vi "古田户外一体站流程自动启动.vi"(11 "参数":T1={"是否启用仪器"=FALSE, "CODMn"={"启动测量模式"={"测量模式"=enum."水样测量"}, "确定按钮"=TRUE}}) -> ()   [LabVIEW 2016, in "PLC.lvlib"]
uses:
  PLC.lvlib
panel:
  out "枚举":enum16{"初始化", "采配水启动", "等待", "配水", "排水", "结束"}(ring)
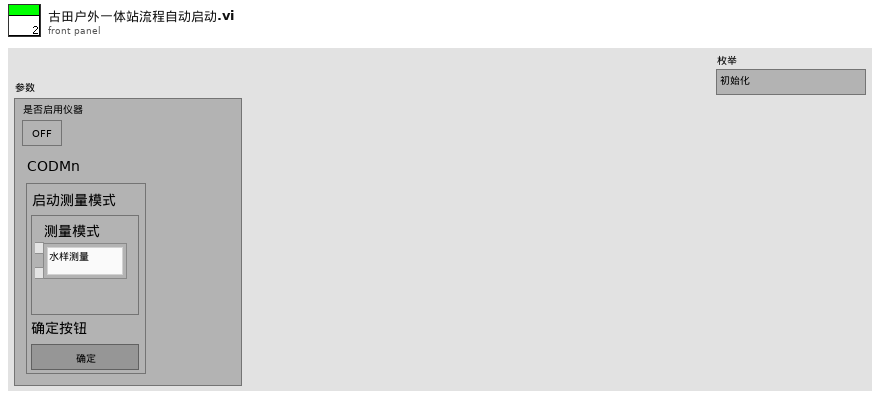
[diagram p1: front panel]
types:
  T1 = cluster{"是否启用仪器":bool, "CODMn":cluster{"启动测量模式":cluster{"测量模式":enum16{"水样测量", "标样核查", "零点核查", "加标回收", "平行样", "校零", "校标"}}, "确定按钮":bool}}
  T2 = cluster{"命令":string, cluster{"starting address":u16, "holding register value":u16}}
  T3 = enum16{"待机", "启动氨氮", "氨氮测量中", "启动总磷", "总磷测量中", "结束"}
  T4 = cluster{"测量模式":enum16{"待机", "水样测试", "标样核查", "零点核查", "跨度核查", "空白测试", "平行样测试", "加标回收", "空白校准", "标样校准", "初始化（清洗）"}, "数据标记表":string, "测量时间":dbl}
  T5 = enum16{"待机", "水样测试", "标样核查", "零点核查", "跨度核查", "空白测试", "平行样测试", "加标回收", "空白校准", "标样校准", "初始化（清洗）"}
  T6 = cluster{"站号":u16, "量程切换":enum32{"H", "L", "AUTO"}, "控制命令":enum16{"启动测量", "标样核查", "零点核查", "跨度核查", "空白测试", "平行样测试", "加标回收", "空白校准", "标样校准", "初始化（清洗）", "停止测试", "仪器重启", "校时", "模式设置", "测量间隔设置", "盲样测试"}, "模式设置":enum16{"待机", "连续模式", "周期模式", "定点模式", "受控模式", "手动模式"}, "测量间隔":u16}
  T7 = cluster{"时间标识":timestamp, "设备":string, "日志信息":string}
  T8 = cluster{"R0":i16, "R1":i16, "R2":i16, "R3":i16, "R4":i16, "R5":i16, "R6":i16, "R7":i16, "R8":i16, "R9":i16, "R10":i16, "R11":i16, "R12":i16, "R13":i16, "R14":i16, "R15":i16, "R16":i16, "R17":i16, "R18":i16, "R19":i16}
  T9 = enum32{"Bad", "Idle", "Run top level", "Running"}
  T10 = cluster{"测量模式":enum16{"水样测量", "标样核查", "零点核查", "加标回收", "平行样", "校零", "校标"}}
  T11 = cluster{"系统时间":timestamp, "工作状态":enum16{"空闲", "水样测试", "标样核查", "零点核查", "跨度核查", "空白测试", "平行样测试", "加标回收", "空白校准", "标样校准", "初始化（清洗）"}, "测量模式":enum16{"待机", "连续模式", "周期模式", "定点模式", "受控模式", "手动模式"}, "告警代码":enum16{"无告警", "缺试剂告警", "缺水样告警", "缺蒸馏水告警", "缺标液告警", "仪表漏液告警", "标定异常告警", "超量程告警", "加热异常", "低试剂预警", "超上限告警", "超下限告警", "仪表内部其他异常", "滴定异常告警", "电极异常告警", "量程切换告警", "参数设置告警", "PH电极电位异常", "电导率电极异常", "浊度光度异常", "溶解氧电极异常", "溶解氧光强异常", "温度异常告警", "PH异常告警", "溶解氧异常告警", "电导率异常告警", "浊度异常告警", "叶绿素异常告警", "藻密度异常告警", "蓝绿藻异常告警", "ORP异常告警", "氨氮异常告警", "清洁刷异常告警", "SD卡异常告警", "蓝牙异常告警", "Wifi异常告警", "流程异常告警"}, "故障代码":enum16{"无故障", "电机故障", "温度故障", "通讯故障", "滴定故障"}, "日志代码":u16, "软件版本":u16, "F0":sgl, "F1":sgl, "F2":sgl, "F3":sgl, "T":sgl, "H":sgl, "id":u16, "flowid":u16, "量程":u16}
  T12 = enum16{"空闲", "水样测试", "标样核查", "零点核查", "跨度核查", "空白测试", "平行样测试", "加标回收", "空白校准", "标样校准", "初始化（清洗）"}
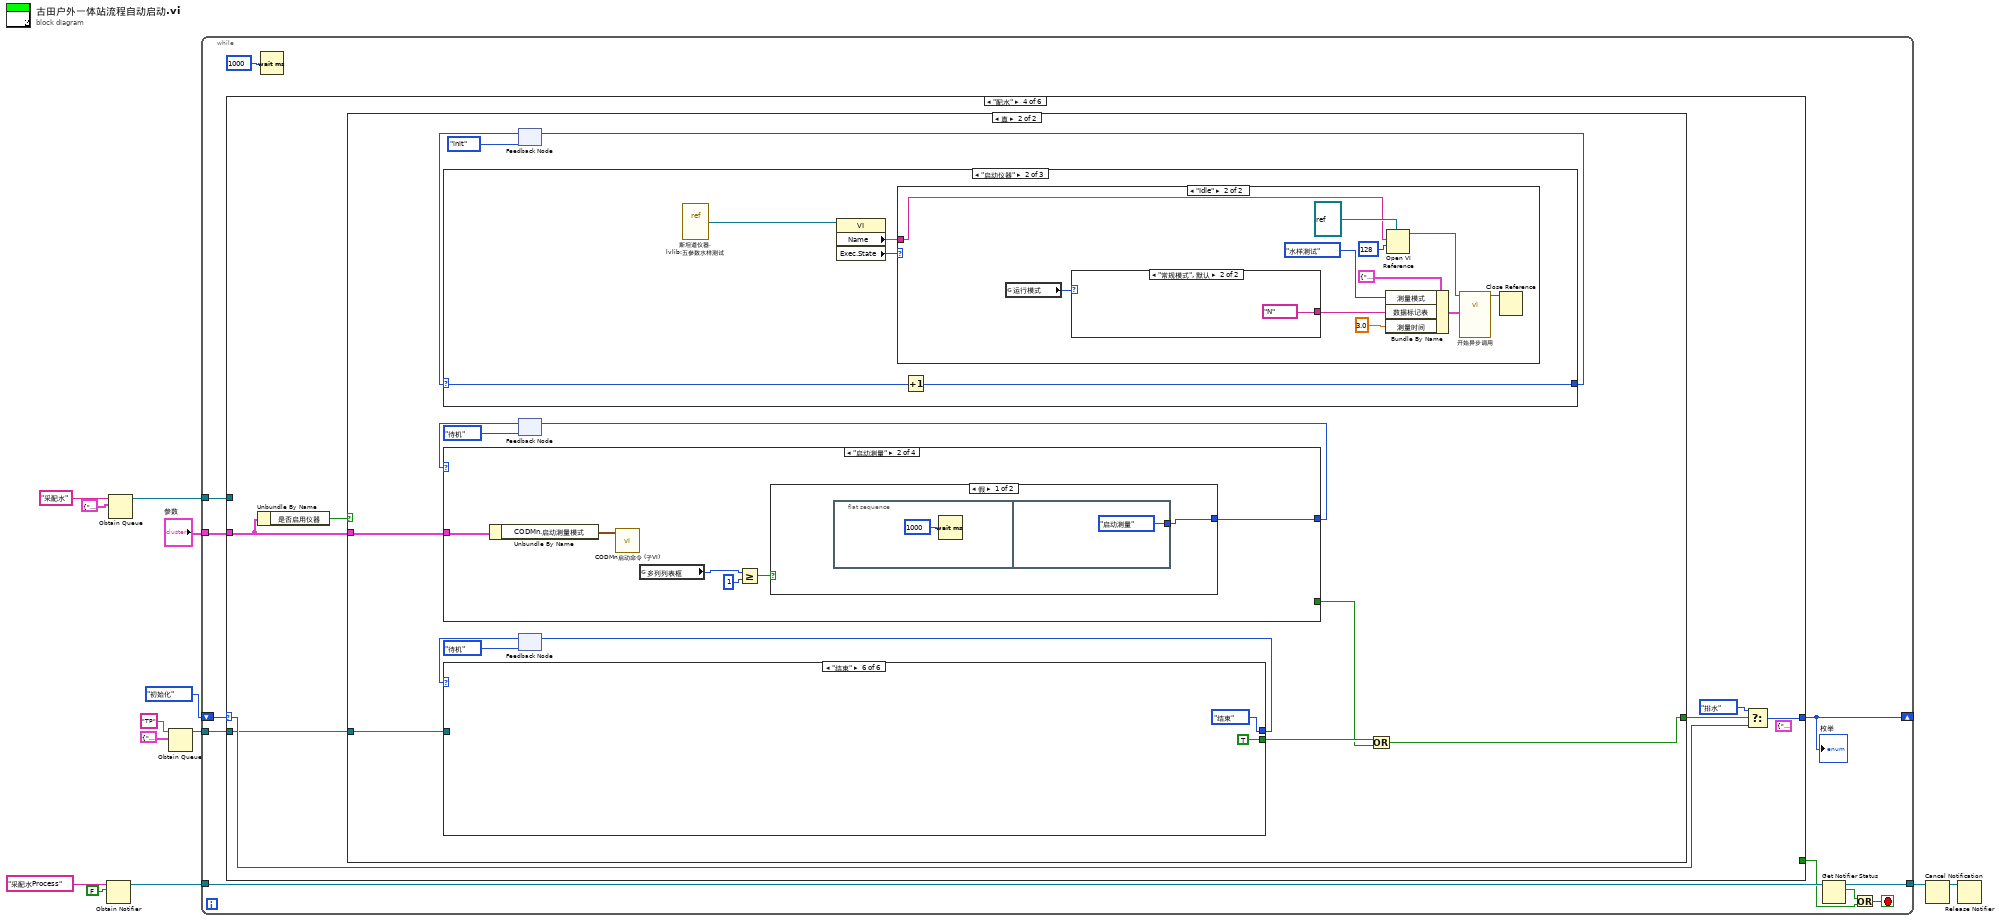
[diagram p0: block diagram]
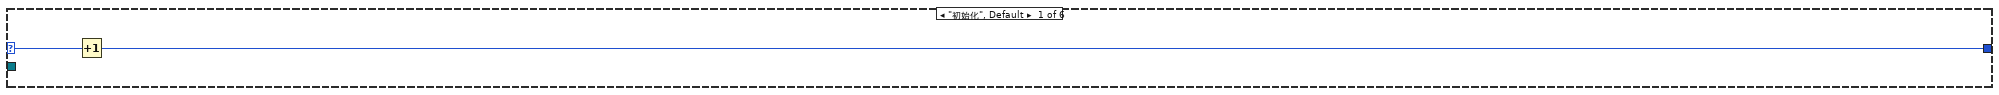
[diagram p2: hidden frame]
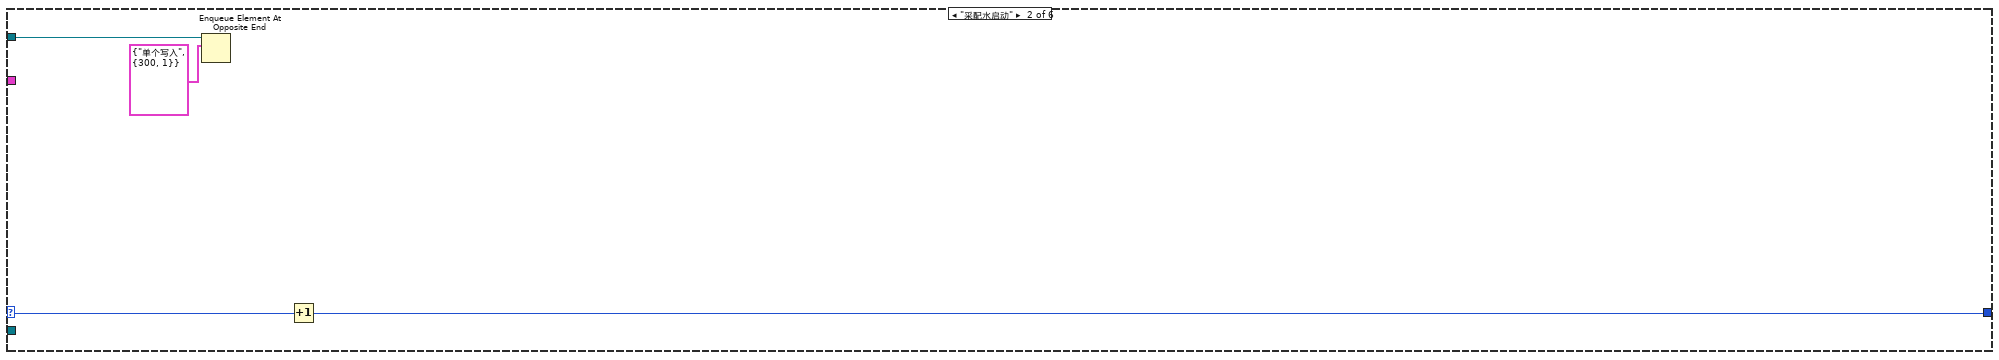
[diagram p3: hidden frame]
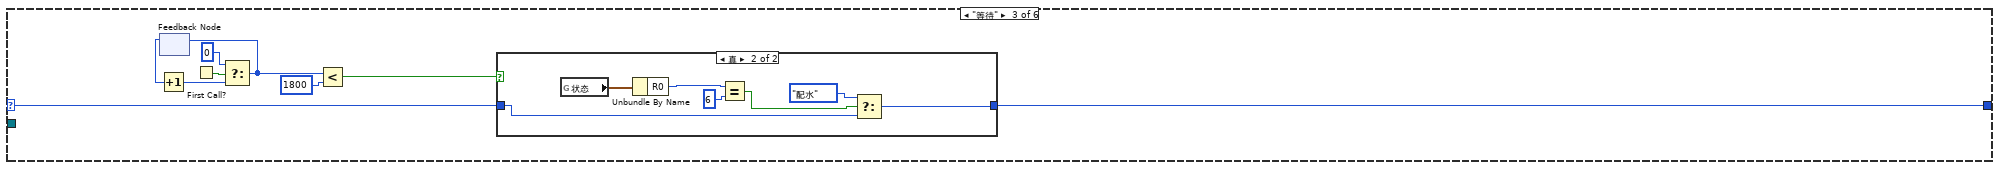
[diagram p4: hidden frame]
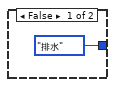
[diagram p5: hidden frame]
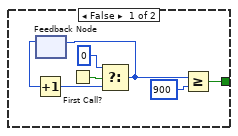
[diagram p6: hidden frame]
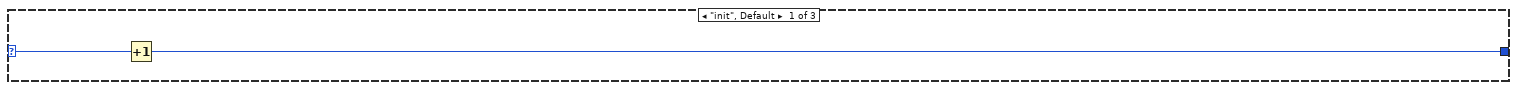
[diagram p7: hidden frame]
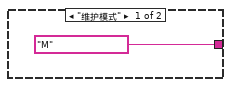
[diagram p9: hidden frame]
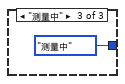
[diagram p10: hidden frame]
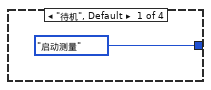
[diagram p11: hidden frame]
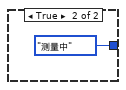
[diagram p12: hidden frame]
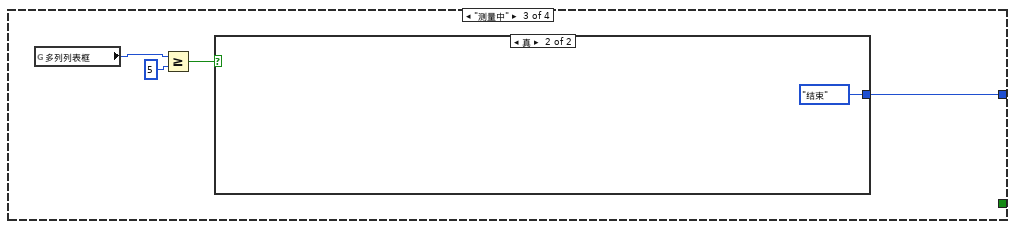
[diagram p13: hidden frame]
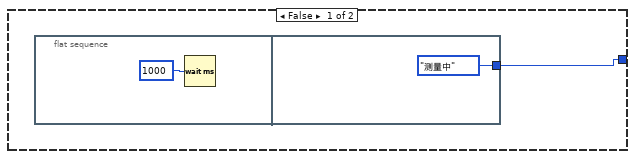
[diagram p14: hidden frame]
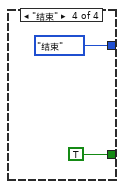
[diagram p15: hidden frame]
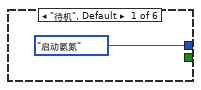
[diagram p16: hidden frame]
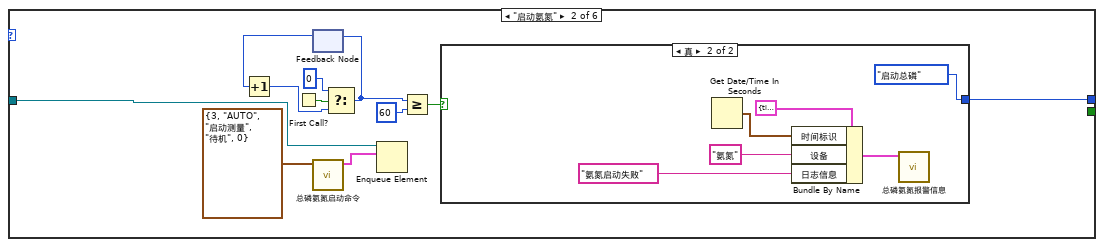
[diagram p17: hidden frame]
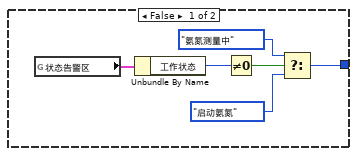
[diagram p18: hidden frame]
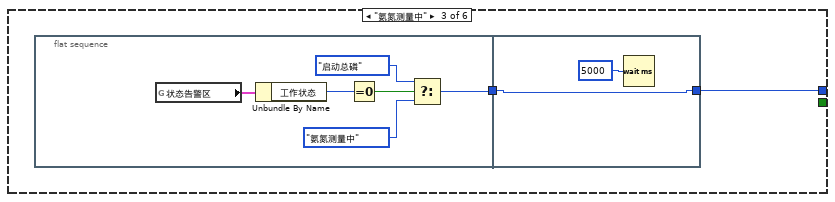
[diagram p19: hidden frame]
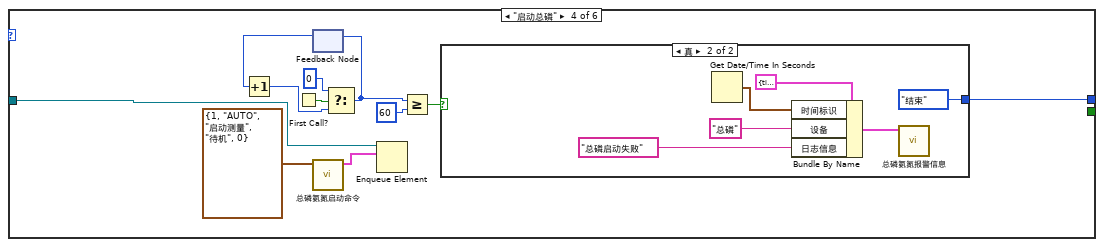
[diagram p20: hidden frame]
diagram:
  n1 = Obtain Notifier(name (unnamed)="采配水Process" ("名称（未命名）"), notification data type=FALSE) -> (notifier out=w3:refnum<notifier>)  [unwired: 2 in, 2 out]
  n2 = Obtain Queue(name (unnamed)="采配水" ("名称（未命名）"), element data type=cluster{"命令":string, "数据":variant} {"命令"="", "数据"=variant}) -> (queue out=w11:refnum<queue>)  [unwired: 3 in, 2 out]
  n3 = Obtain Queue(name (unnamed)="TP" ("名称（未命名）"), element data type=cluster{"命令":string, "data":variant} {"命令"="", "data"=variant}) -> (queue out=w7:refnum<queue>)  [unwired: 3 in, 2 out]
  n4 = while {
    tunnel: w11 -> [w24]
    shift-right: [w22] -> _
    shift-left: enum16{"初始化", "采配水启动", "等待", "配水", "排水", "结束"}."初始化" ("枚举") -> [w23]
    tunnel: w7 -> [w20]
    tunnel: "参数" -> [w19]
    tunnel: w3 -> [w18]
    tunnel: [w17] -> w2
    stop <- w16 stop-if-true
    n5 = case shown="\"配水\"" w23 {
      selector: w23 -> [w26 w28 w37 w53 w188 w193]
      tunnel: w24 -> [_ w29 _ _ w189 _]
      tunnel: [w25 w27 w36 w52 w187 w192] -> w22
      tunnel: [_ _ _ _ _ TRUE] -> w15
      tunnel: w20 -> [_ _ _ w51 _ _]
      tunnel: w19 -> [_ _ _ w48 _ _]
      frame "初始化", Default {
        n6 = Increment(x=w26) -> (x+1=w25:enum16{"初始化", "采配水启动", "等待", "配水", "排水", "结束"})
      }
      frame "采配水启动" {
        n7 = Enqueue Element At Opposite End(queue=w29, element=T2 {"命令"="单个写入", {"starting address"=300, "holding register value"=1}} ("元素")) -> ()  [unwired: 2 in, 3 out]
        n8 = Increment(x=w28) -> (x+1=w27:enum16{"初始化", "采配水启动", "等待", "配水", "排水", "结束"})
      }
      frame "等待" {
        n9 = feedback #1() -> (w33:i32)  [unwired: 1 in]
        n10 = Increment(x=w33) -> (x+1=w32:i32)
        n11 = First Call?() -> (First Call?: T/F=w34:bool)
        n12 = Select(t=0, s=w34, f=w32) -> (s? t:f=w31:i32)
        n13 = feedback-in #1(w31) -> ()
        n14 = Less?(x=w31, y=1800) -> (x < y?=w38:bool)
        n15 = case shown="真" w38 {
          tunnel: w37 -> [_ w42]
          tunnel: [enum16{"初始化", "采配水启动", "等待", "配水", "排水", "结束"}."排水" ("枚举") w41] -> w36
          frame False {
          }
          frame True {
            n16 = global read "采配水全局变量.vi" "状态"() -> (w47:T8)
            n17 = Unbundle By Name(w47) -> ("R0"=w46:i16)
            n18 = Equal?(x=w46, y=i16 6) -> (x = y?=w44:bool)
            n19 = Select(t=enum16{"初始化", "采配水启动", "等待", "配水", "排水", "结束"}."配水" ("枚举"), s=w44, f=w42) -> (s? t:f=w41:enum16{"初始化", "采配水启动", "等待", "配水", "排水", "结束"})
          }
        }
      }
      frame "配水" {
        (unwired) cluster{"命令":string, "data":variant} {"命令"="启动", "data"=variant(cluster{"站号":u16, "控制命令输出":u16[]} {"站号"=1, "控制命令输出"=[256, 0]})} ("元素")
        n20 = Unbundle By Name(w48) -> ("是否启用仪器"=w50:bool)
        n21 = case shown="真" w50 {
          tunnel: w51 -> [_ w72]
          tunnel: [w55 w65] -> w49
          tunnel: w48 -> [_ w68]
          frame False {
            n22 = feedback #2() -> (w59:i32)  [unwired: 1 in]
            n23 = Increment(x=w59) -> (x+1=w58:i32)
            n24 = First Call?() -> (First Call?: T/F=w60:bool)
            n25 = Select(t=0, s=w60, f=w58) -> (s? t:f=w56:i32)
            n26 = feedback-in #2(w56) -> ()
            n27 = Greater Or Equal?(x=w56, y=900) -> (x >= y?=w55:bool)
          }
          frame True {
            n28 = feedback #3(enum16{"init", "启动仪器", "测量中"}."init") -> (w63:enum16{"init", "启动仪器", "测量中"})
            n29 = case shown="\"启动仪器\"" w63 {
              selector: w63 -> [w77 w82 _]
              tunnel: [w76 w81 enum16{"init", "启动仪器", "测量中"}."测量中"] -> w64
              frame "init", Default {
                n30 = Increment(x=w77) -> (x+1=w76:enum16{"init", "启动仪器", "测量中"})
              }
              frame "启动仪器" {
                n31 = vi-ref "斯坦道仪器.lvlib:五参数水样测试.vi"() -> (w79:refnum<vi>)
                n32 = property class="VI"(reference=w79) -> ("Name"=w78:string, "Exec.State"=w80:T9)  [unwired: 1 in, 2 out]
                n33 = case shown="\"Idle\"" w80 {
                  tunnel: w78 -> [_ w89]
                  frame "Bad", Default {
                  }
                  frame "Idle" {
                    n34 = global read "系统变量.vi" "运行模式"() -> (w84:enum16{"维护模式", "常规模式", "应急模式", "质控模式"})
                    n35 = case shown="\"常规模式\", 默认" w84 {
                      tunnel: ["M" ("数据标记表") "N" ("数据标记表")] -> w83
                      frame "维护模式" {
                      }
                      frame "常规模式", Default {
                      }
                    }
                    n36 = Bundle By Name(cluster=T4 {"测量模式"=enum."待机", "数据标记表"="", "测量时间"=0.0} ("启动参数"), "测量模式"=T5."水样测试", "数据标记表"=w83, "测量时间"=3.0) -> (w85:T4)
                    n37 = Open VI Reference(type specifier VI Refnum (for type only)=refnum<vi> refnum ("类型说明符VI引用句柄（仅用于类型）"), vi path=w89, options=128 ("选项")) -> (vi reference=w88:refnum<vi>)  [unwired: 3 in, 1 out]
                    n38 = call-by-ref "开始异步调用"(reference=w88, "启动参数"=w85) -> (reference out=w87:refnum<vi>)  [unwired: 12 in, 1 out]
                    n39 = Close Reference(reference=w87) -> ()  [unwired: 1 in, 1 out]
                  }
                }
                n40 = Increment(x=w82) -> (x+1=w81:enum16{"init", "启动仪器", "测量中"})
              }
              frame "测量中" {
              }
            }
            n41 = feedback-in #3(w64) -> ()
            n42 = feedback #4(enum16{"待机", "启动测量", "测量中", "结束"}."待机") -> (w70:enum16{"待机", "启动测量", "测量中", "结束"})
            n43 = case shown="\"启动测量\"" w70 {
              tunnel: [enum16{"待机", "启动测量", "测量中", "结束"}."启动测量" w100 w109 enum16{"待机", "启动测量", "测量中", "结束"}."结束"] -> w69
              tunnel: w68 -> [_ w103 _ _]
              tunnel: [_ _ _ TRUE] -> w66
              frame "待机", Default {
              }
              frame "启动测量" {
                n44 = Unbundle By Name(w103) -> ("CODMn.启动测量模式"=w98:T10)
                n45 = call "CODMn启动命令 (子VI).vi"("启动测量模式"=w98) -> ()  [unwired: 11 in]
                n46 = global read "运行时序全局变量.vi" "多列列表框"() -> (w99:i32)
                n47 = Greater Or Equal?(x=w99, y=1) -> (x >= y?=w101:bool)
                n48 = case shown="假" w101 {
                  tunnel: [w104 enum16{"待机", "启动测量", "测量中", "结束"}."测量中"] -> w100
                  frame False {
                    n49 = flat-sequence {
                      tunnel: [enum16{"待机", "启动测量", "测量中", "结束"}."启动测量"] -> w104
                      frame #0 {
                        n50 = Wait (ms)(milliseconds to wait=u32 1000 ("等待时间（毫秒）")) -> ()  [unwired: 1 out]
                      }
                      frame #1 {
                      }
                    }
                  }
                  frame True {
                  }
                }
              }
              frame "测量中" {
                n51 = global read "运行时序全局变量.vi" "多列列表框"() -> (w108:i32)
                n52 = Greater Or Equal?(x=w108, y=5) -> (x >= y?=w110:bool)
                n53 = case shown="真" w110 {
                  tunnel: [w112 enum16{"待机", "启动测量", "测量中", "结束"}."结束"] -> w109
                  frame False {
                    n54 = flat-sequence {
                      tunnel: [enum16{"待机", "启动测量", "测量中", "结束"}."测量中"] -> w112
                      frame #0 {
                        n55 = Wait (ms)(milliseconds to wait=u32 1000 ("等待时间（毫秒）")) -> ()  [unwired: 1 out]
                      }
                      frame #1 {
                      }
                    }
                  }
                  frame True {
                  }
                }
              }
              frame "结束" {
              }
            }
            n56 = feedback-in #4(w69) -> ()
            n57 = feedback #5(T3."待机") -> (w74:T3)
            n58 = case shown="\"结束\"" w74 {
              tunnel: [T3."启动氨氮" w128 w143 w161 w176 T3."结束"] -> w73
              tunnel: w72 -> [_ w129 _ w162 _ _]
              tunnel: [_ _ _ _ _ TRUE] -> w67
              frame "待机", Default {
              }
              frame "启动氨氮" {
                n59 = First Call?() -> (First Call?: T/F=w126:bool)
                n60 = feedback #6() -> (w125:i32)  [unwired: 1 in]
                n61 = Increment(x=w125) -> (x+1=w124:i32)
                n62 = call "总磷氨氮启动命令.vi"("参数"=T6 {"站号"=3, "量程切换"=enum."AUTO", "控制命令"=enum."启动测量", "模式设置"=enum."待机", "测量间隔"=0}) -> ("启动命令"=w120:cluster{"命令":string, "data":variant})  [unwired: 10 in]
                n63 = Select(t=0, s=w126, f=w124) -> (s? t:f=w123:i32)
                n64 = feedback-in #6(w123) -> ()
                n65 = Enqueue Element(queue=w129, element=w120) -> ()  [unwired: 2 in, 3 out]
                n66 = Greater Or Equal?(x=w123, y=60) -> (x >= y?=w121:bool)
                n67 = case shown="真" w121 {
                  tunnel: [w132 T3."启动总磷"] -> w128
                  frame False {
                    n68 = global read "VAR总磷氨氮全局变量.vi" "状态告警区"() -> (w135:T11)
                    n69 = Unbundle By Name(w135) -> ("工作状态"=w134:T12)
                    n70 = Not Equal To 0?(x=w134) -> (x != 0?=w133:bool)
                    n71 = Select(t=T3."氨氮测量中", s=w133, f=T3."启动氨氮") -> (s? t:f=w132:T3)
                  }
                  frame True {
                    n72 = Get Date/Time In Seconds() -> (seconds since 1Jan1904=w140:timestamp)
                    n73 = Bundle By Name(cluster=T7 {"时间标识"=timestamp(0 s since 1904-01-01), "设备"="", "日志信息"=""} ("data in"), "时间标识"=w140, "设备"="氨氮", "日志信息"="氨氮启动失败") -> (w136:T7)
                    n74 = call "总磷氨氮报警信息.vi"("data in"=w136) -> ()  [unwired: 11 in]
                  }
                }
              }
              frame "氨氮测量中" {
                n75 = flat-sequence {
                  tunnel: [w147] -> w142
                  tunnel: [w151] -> w143
                  tunnel: w142 -> [w151]
                  frame #0 {
                    n76 = global read "VAR总磷氨氮全局变量.vi" "状态告警区"() -> (w148:T11)
                    n77 = Unbundle By Name(w148) -> ("工作状态"=w149:T12)
                    n78 = Equal To 0?(x=w149) -> (x = 0?=w146:bool)
                    n79 = Select(t=T3."启动总磷", s=w146, f=T3."氨氮测量中") -> (s? t:f=w147:T3)
                  }
                  frame #1 {
                    n80 = Wait (ms)(milliseconds to wait=u32 5000 ("等待时间（毫秒）")) -> ()  [unwired: 1 out]
                  }
                }
              }
              frame "启动总磷" {
                n81 = First Call?() -> (First Call?: T/F=w159:bool)
                n82 = feedback #7() -> (w158:i32)  [unwired: 1 in]
                n83 = Increment(x=w158) -> (x+1=w157:i32)
                n84 = call "总磷氨氮启动命令.vi"("参数"=T6 {"站号"=1, "量程切换"=enum."AUTO", "控制命令"=enum."启动测量", "模式设置"=enum."待机", "测量间隔"=0}) -> ("启动命令"=w153:cluster{"命令":string, "data":variant})  [unwired: 10 in]
                n85 = Select(t=0, s=w159, f=w157) -> (s? t:f=w156:i32)
                n86 = feedback-in #7(w156) -> ()
                n87 = Enqueue Element(queue=w162, element=w153) -> ()  [unwired: 2 in, 3 out]
                n88 = Greater Or Equal?(x=w156, y=60) -> (x >= y?=w154:bool)
                n89 = case shown="真" w154 {
                  tunnel: [w165 T3."结束"] -> w161
                  frame False {
                    n90 = global read "VAR总磷氨氮全局变量.vi" "状态告警区"() -> (w166:T11)
                    n91 = Unbundle By Name(w166) -> ("工作状态"=w167:T12)
                    n92 = Not Equal To 0?(x=w167) -> (x != 0?=w168:bool)
                    n93 = Select(t=T3."总磷测量中", s=w168, f=T3."启动总磷") -> (s? t:f=w165:T3)
                  }
                  frame True {
                    n94 = Get Date/Time In Seconds() -> (seconds since 1Jan1904=w174:timestamp)
                    n95 = Bundle By Name(cluster=T7 {"时间标识"=timestamp(0 s since 1904-01-01), "设备"="", "日志信息"=""} ("data in"), "时间标识"=w174, "设备"="总磷", "日志信息"="总磷启动失败") -> (w169:T7)
                    n96 = call "总磷氨氮报警信息.vi"("data in"=w169) -> ()  [unwired: 11 in]
                  }
                }
              }
              frame "总磷测量中" {
                n97 = flat-sequence {
                  tunnel: [w180] -> w175
                  tunnel: [w184] -> w176
                  tunnel: w175 -> [w184]
                  frame #0 {
                    n98 = global read "VAR总磷氨氮全局变量.vi" "状态告警区"() -> (w181:T11)
                    n99 = Unbundle By Name(w181) -> ("工作状态"=w182:T12)
                    n100 = Equal To 0?(x=w182) -> (x = 0?=w179:bool)
                    n101 = Select(t=T3."结束", s=w179, f=T3."总磷测量中") -> (s? t:f=w180:T3)
                  }
                  frame #1 {
                    n102 = Wait (ms)(milliseconds to wait=u32 5000 ("等待时间（毫秒）")) -> ()  [unwired: 1 out]
                  }
                }
              }
              frame "结束" {
              }
            }
            n103 = feedback-in #5(w73) -> ()
            n104 = Or(x=w67, y=w66) -> (x .or. y?=w65:bool)
          }
        }
        n105 = Select(t=enum16{"初始化", "采配水启动", "等待", "配水", "排水", "结束"}."排水" ("枚举"), s=w49, f=w53) -> (s? t:f=w52:enum16{"初始化", "采配水启动", "等待", "配水", "排水", "结束"})
      }
      frame "排水" {
        n106 = Enqueue Element At Opposite End(queue=w189, element=T2 {"命令"="单个写入", {"starting address"=303, "holding register value"=1}} ("元素")) -> ()  [unwired: 2 in, 3 out]
        n107 = Increment(x=w188) -> (x+1=w187:enum16{"初始化", "采配水启动", "等待", "配水", "排水", "结束"})
      }
      frame "结束" {
        n108 = Increment(x=w193) -> (x+1=w192:enum16{"初始化", "采配水启动", "等待", "配水", "排水", "结束"})
      }
    }
    "枚举" <- w22
    n109 = Wait (ms)(milliseconds to wait=u32 1000 ("等待时间（毫秒）")) -> ()  [unwired: 1 out]
    n110 = Get Notifier Status(notifier=w18) -> (notifier out=w17:refnum<notifier>, current notification=w14:bool)  [unwired: 1 in, 3 out]
    n111 = Or(x=w14, y=w15) -> (x .or. y?=w16:bool)
  }
  n112 = Cancel Notification(0:w2) -> (8:w1:refnum<notifier>)  [unwired: 1 in, 2 out]
  n113 = Release Notifier(notifier=w1) -> ()  [unwired: 2 in, 3 out]
